vi "Read Current Max.vi"(0 "VISA resource name":refnum<visa-resource-name>, 11 "error in (no error)":errorcluster) -> (4 "VISA resource name out":refnum<visa-resource-name>, 6 "Current Max":string, 15 "error out":errorcluster)   [LabVIEW 2020, in "eec EST 300.lvlib"]
doc: "RDM? \nRead Current Max."
uses:
  <instrlib>/eec EST 300/eec EST 300.lvlib
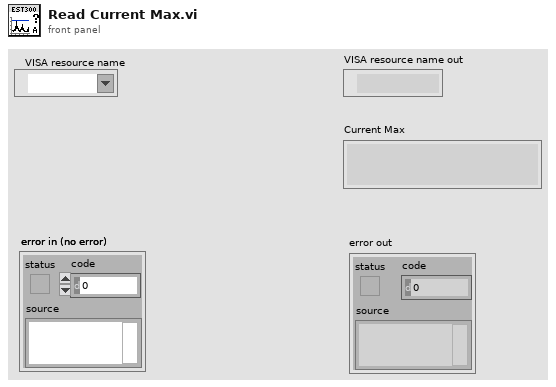
[diagram p1: front panel]
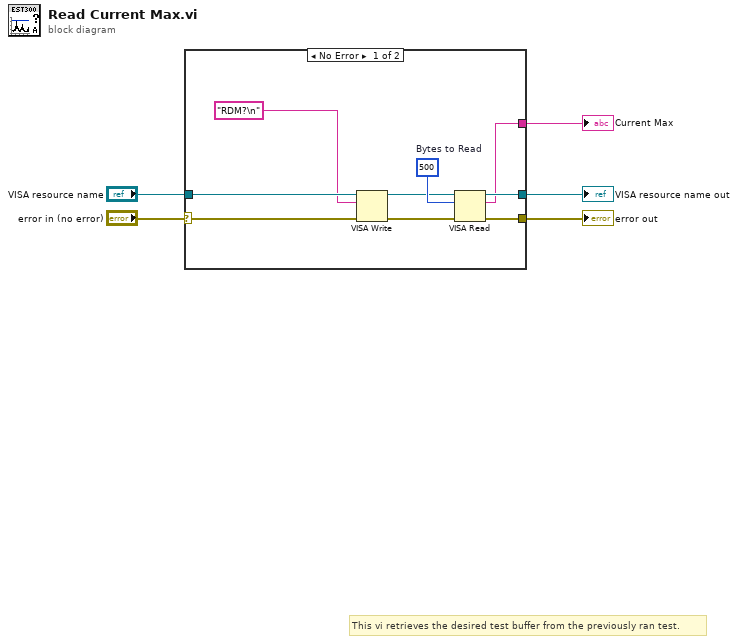
[diagram p0: block diagram]
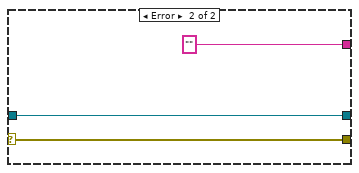
[diagram p2: hidden frame]
diagram:
  # "This vi retrieves the desired test buffer from the previously ran test."
  n1 = case shown="No Error" "error in (no error)" {
    selector: "error in (no error)" -> [w14 w17]
    tunnel: [w12 w17] -> w4
    tunnel: [w11 w16] -> w2
    tunnel: "VISA resource name" -> [w13 w16]
    tunnel: [w10 "" ("Decoded Response")] -> w1
    frame No Error {
      w9 = u32 500  # Bytes to Read
      n2 = VISA Write(VISA resource name=w13, write buffer="RDM?\n" ("string (\"\")"), error in (no error)=w14) -> (VISA resource name out=w7:refnum<visa-resource-name>, error out=w8:errorcluster)  [unwired: 1 out]
      n3 = VISA Read(VISA resource name=w7, byte count=w9, error in (no error)=w8) -> (VISA resource name out=w11:refnum<visa-resource-name>, read buffer=w10:string, error out=w12:errorcluster)  [unwired: 1 out]
    }
    frame Error {
    }
  }
  "error out" <- w4
  "VISA resource name out" <- w2
  "Current Max" <- w1
